vi "VecBuilder_5x1Fill.vi"(6 "R4":dbl, 8 "R3":dbl, 9 "R2":dbl, 10 "R1":dbl, 11 "R0":dbl) -> (3 "output matrix":T1)   [LabVIEW 2019, in "Trajectory_Library.lvlib"]
doc: "Build a 5 x 1 Matrix (vector) from an array of input values.\n\nInputs:\n -- R0 -- Input value 1\n -- R1 -- Input value 2\n -- R2 -- Input value 3\n -- R3 -- Input value 4\n -- R4 -- Input value 5\n\nOutputs:\n -- Output Matrix -- Resulting 5 x 1 matrix (vector)"
uses:
  Trajectory_Library.lvlib
  <vilib>/Analysis/Matrix/Datatypes/RealMatrix.ctl
  <vilib>/Analysis/Matrix/NI_Matrix.lvlib
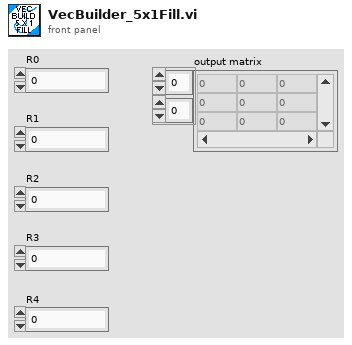
[diagram p1: front panel]
types:
  T1 = typedef "NI_Matrix.lvlib/RealMatrix.ctl" = dbl[][]
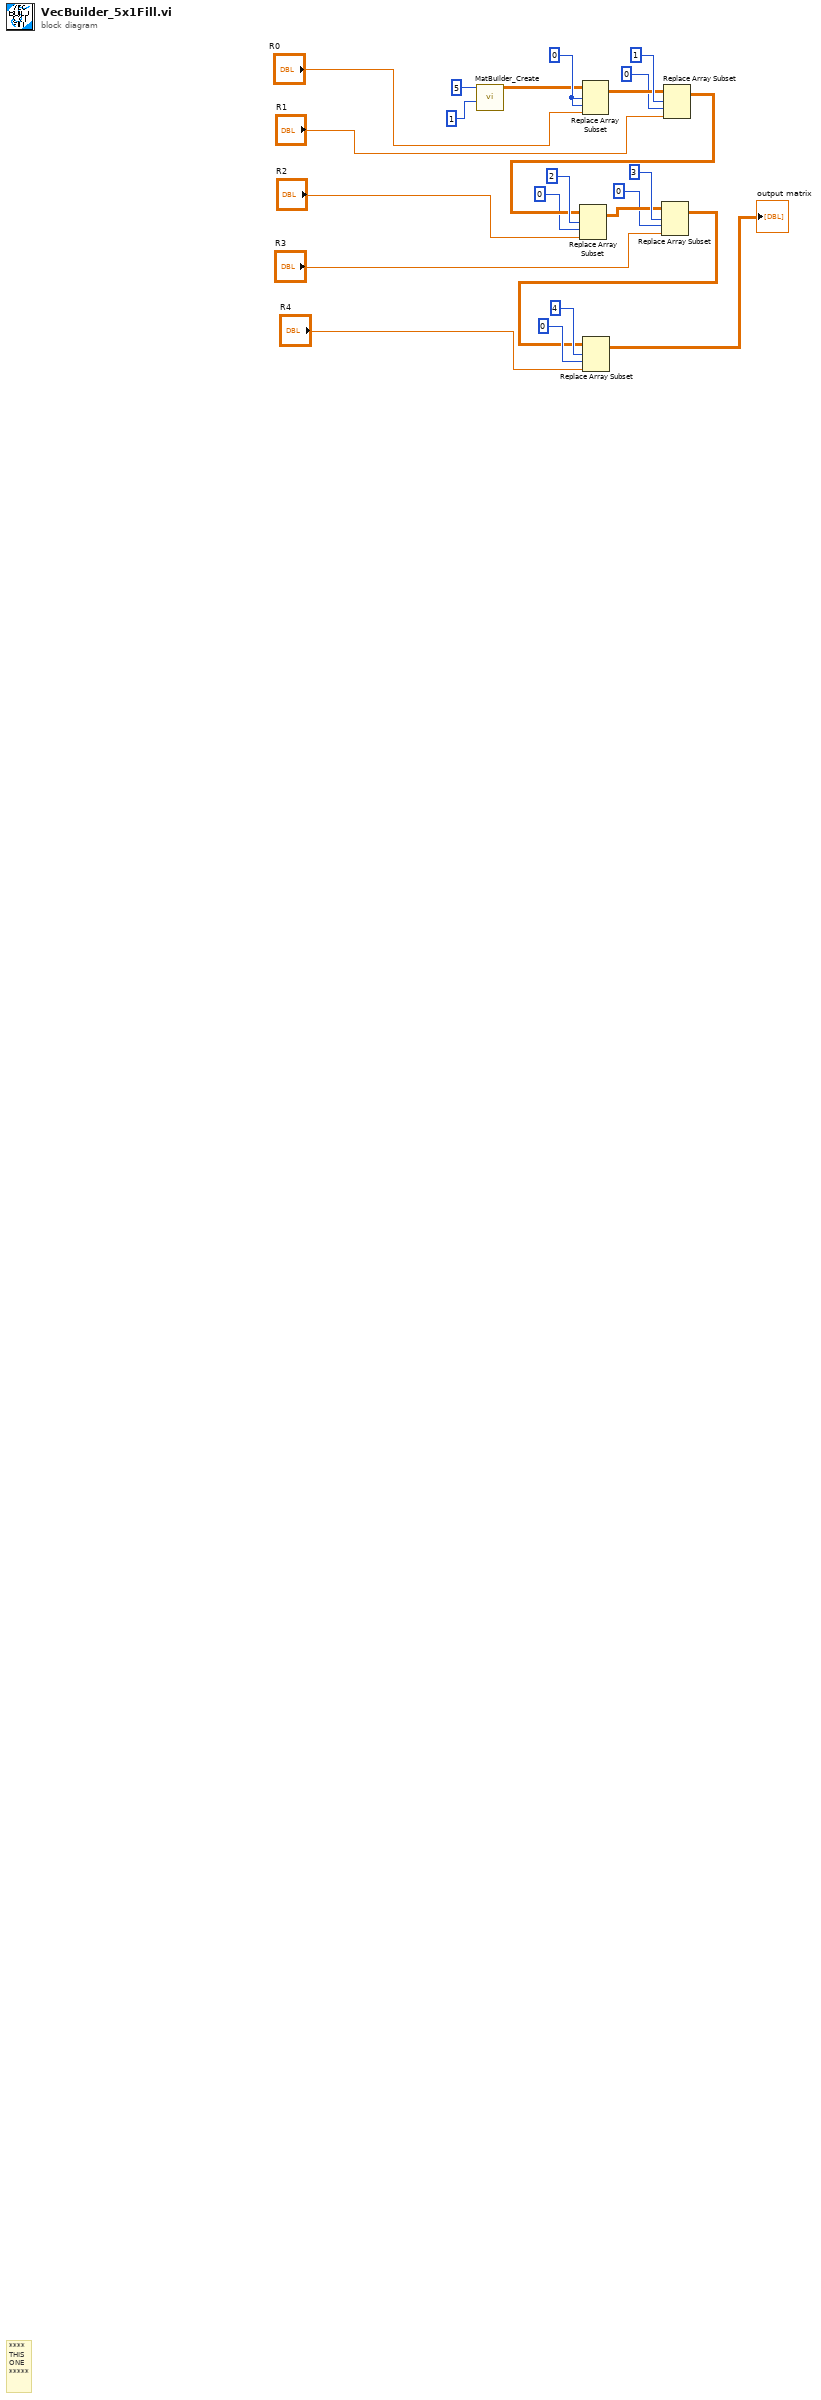
[diagram p0: block diagram]
diagram:
  w22 = 0 ("index (col)")
  # "****\nTHIS\nONE\n*****"
  n1 = call "MatBuilder_Create.vi"("Columns"=1, "Rows"=5) -> ("output matrix"=w14:T1)  [unwired: 9 in]
  n2 = Replace Array Subset(array=w14, new element="R0", index (row)=w22, index (col)=w22) -> (w20:T1)
  n3 = Replace Array Subset(array=w20, new element="R1", index (row)=1 ("index (col)"), index (col)=0 ("disabled index (col)")) -> (w11:T1)
  n4 = Replace Array Subset(array=w11, new element="R2", index (row)=2 ("index (col)"), index (col)=0 ("disabled index (col)")) -> (w10:T1)
  n5 = Replace Array Subset(array=w10, new element="R3", index (row)=3 ("index (col)"), index (col)=0 ("disabled index (col)")) -> (w3:T1)
  n6 = Replace Array Subset(array=w3, new element="R4", index (row)=4 ("index (col)"), index (col)=0 ("disabled index (col)")) -> (→"output matrix":T1)
